vi "Calc.vi"(4 "Обратный коэффицент делителя напряжения, Безразм":dbl, 6 "Сопротивление шунта, Ом":dbl, 7 "0 in":i32, 9 "Опорное напряжение АЦП, Вольты":dbl, 10 "Разрядность АЦП":u8, 11 "1 in":i32) -> (2 "Numeric 2":dbl, 3 "Numeric":dbl)   [LabVIEW 2013]
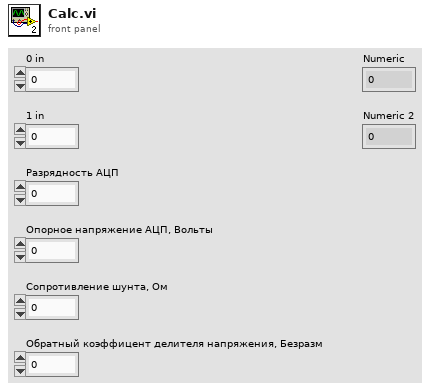
[diagram p1: front panel]
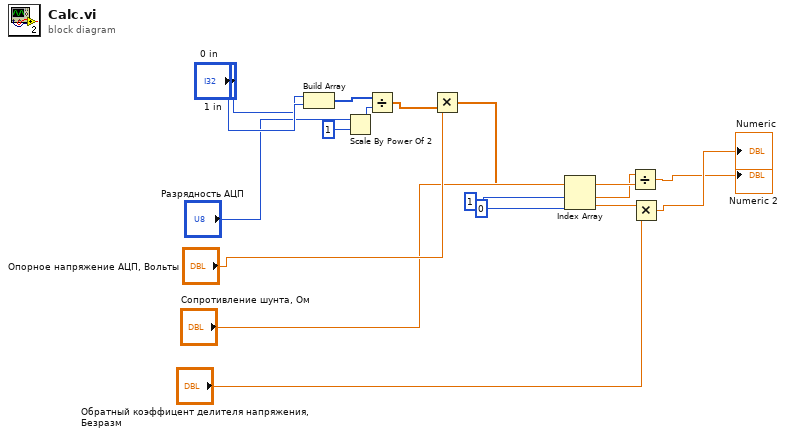
[diagram p0: block diagram]
diagram:
  n1 = Build Array("0 in", "1 in") -> (w15:i32[])
  n2 = Scale By Power Of 2(n="Разрядность АЦП", x=1) -> (x*2^n=w1:i32)
  n3 = Divide(x=w15, y=w1) -> (x/y=w4:dbl[])
  n4 = Multiply(x="Опорное напряжение АЦП, Вольты", y=w4) -> (x*y=w5:dbl[])
  n5 = Index Array(array=w5, index #1=1, index #2=0) -> (element #1=w9:dbl, element #2=w8:dbl)
  n6 = Divide(x=w9, y="Сопротивление шунта, Ом") -> (x/y=→"Numeric 2":dbl)
  n7 = Multiply(x=w8, y="Обратный коэффицент делителя напряжения, Безразм") -> (x*y=→"Numeric":dbl)
